vi "dfd_FXP Direct IIR II Transposed with IS.vi"(6 "state in":i64[](array[numeric]), 7 "quantizers":T5[](array[typedef]) {"source" items=["Coef a/k"=0, "Coef b/v"=7, "Input"=1, "Output"=2, "Multiplicand"=3, "Product"=4, "Sum"=5, "Delay"=6, "Gain"=8]}, 8 "filtering statistics in":T4(array[cluster]) {"statistics information"."min value" format="%.2f"; "statistics information"."max value" format="%.2f"; "Quantizer Source" items=["Coefficients a/k"=0, "Coefficients b/v"=7, "Input"=1, "Output"=2, "Multiplicand"=3, "Product"=4, "Sum"=5, "Delay"=6]}, 9 "coef a":T7, 10 "coef b":T7, 11 "X":T7) -> (0 "filtering statistics out":T4(array[cluster]) {"statistics information"."min value" format="%.2f"; "statistics information"."max value" format="%.2f"; "Quantizer Source" items=["Coefficients a/k"=0, "Coefficients b/v"=7, "Input"=1, "Output"=2, "Multiplicand"=3, "Product"=4, "Sum"=5, "Delay"=6]}, 3 "filtered X":T7, 4 "state out":i64[](array[numeric]))   [LabVIEW 2017, in "NI_DigFilter_FXP.lvlib"]
uses:
  <vilib>/addons/Digital Filter Design/NI_DigFilter_FXP.lvlib
  <vilib>/addons/Digital Filter Design/_Objects.llb/dfd_DFXP Data Type (vector).ctl
  <vilib>/addons/Digital Filter Design/_Objects.llb/dfd_DFXP Operation Parameter.ctl
  <vilib>/addons/Digital Filter Design/_Objects.llb/dfd_Internal Quantization Srcs.ctl
  <vilib>/addons/Digital Filter Design/_Objects.llb/DFD Quantization Sources.ctl
  <vilib>/addons/Digital Filter Design/_Objects.llb/DFD FXP Statistics Data.ctl
  <vilib>/addons/Digital Filter Design/_Objects.llb/dfd_DFXP Data Type (scaler).ctl
  <vilib>/addons/Digital Filter Design/NI_DigFilterLicensed.lvlib
panel:
  in  "DFXP Value":T1={"value"=0, "wl"=0, "iwl"=0, "Signed"=TRUE} {"value" format="%.0x"}
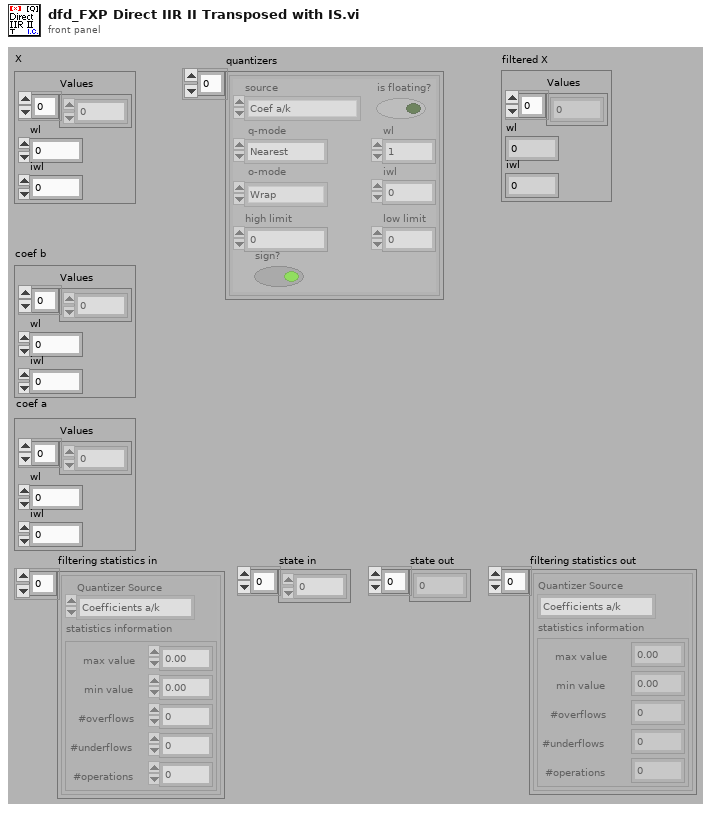
[diagram p1: front panel]
types:
  T1 = typedef "dfd_DFXP Data Type (scaler).ctl" = cluster{"value":i64, "wl":i16, "iwl":i16, "Signed":bool}
  T2 = typedef "NI_DigFilterLicensed.lvlib/DFD Quantization Sources.ctl" = u16
  T3 = typedef "NI_DigFilterLicensed.lvlib/DFD FXP Statistics Data.ctl" = cluster{"max value":ext, "min value":ext, "#overflows":i32, "#underflows":i32, "#operations":i32}
  T4 = cluster{"Quantizer Source":T2, "statistics information":T3}[]
  T5 = typedef "dfd_DFXP Operation Parameter.ctl" = cluster{"source":T6, "is floating?":bool, "o-mode":enum16{"Saturation", "Wrap"}, "q-mode":enum16{"Nearest", "Truncation"}, "wl":i16, "high limit":i64, "low limit":i64, "iwl":i16, "sign?":bool}
  T6 = typedef "NI_DigFilterLicensed.lvlib/dfd_Internal Quantization Srcs.ctl" = u16
  T7 = typedef "dfd_DFXP Data Type (vector).ctl" = cluster{"Values":i64[], "wl":i16, "iwl":i16}
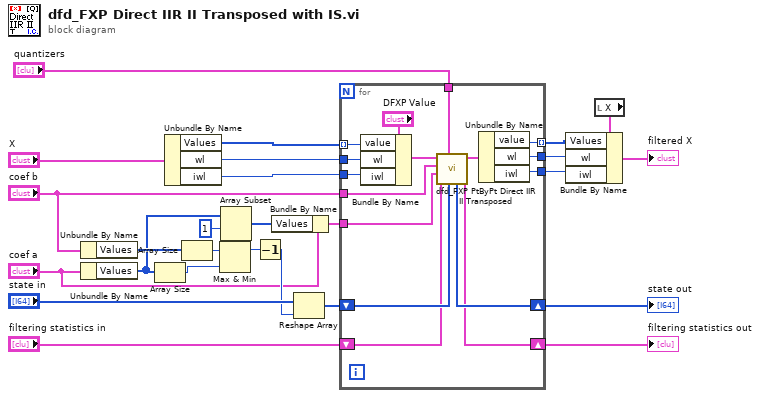
[diagram p0: block diagram]
diagram:
  n1 = Unbundle By Name("coef b") -> ("Values"=w11:i64[])
  n2 = Unbundle By Name("coef a") -> ("Values"=w10:i64[])
  n3 = Array Size(array=w10) -> (size(s)=w24:i32)
  n4 = Unbundle By Name("X") -> ("Values"=w7:i64[], "wl"=w6:i16, "iwl"=w5:i16)
  n5 = Array Size(array=w11) -> (size(s)=w23:i32)
  n6 = Max & Min(x=w23, y=w24) -> (max(x,y)=w21:i32)  [unwired: 1 out]
  n7 = Array Subset(array=w10, index=1) -> (w19:i64[])  [unwired: 1 in]
  n8 = Decrement(x=w21) -> (x-1=w14:i32)
  n9 = Bundle By Name(cluster="coef a", "Values"=w19) -> (w9:T7)
  n10 = Reshape Array("state in", w14) -> (w22:i64[])
  n11 = for {
    tunnel: w7 -> [w42] mode=indexing
    shift-right: [w36] -> w18
    shift-left: w22 -> [w37]
    tunnel: w9 -> [w39]
    tunnel: "coef b" -> [w40]
    tunnel: [w29] -> w16 mode=indexing
    tunnel: "quantizers" -> [w38]
    shift-right: [w34] -> w12
    shift-left: "filtering statistics in" -> [w35]
    tunnel: w6 -> [w31]
    tunnel: w5 -> [w30]
    tunnel: [w28] -> w2
    tunnel: [w27] -> w1
    n12 = Bundle By Name(cluster="DFXP Value", "value"=w42, "wl"=w31, "iwl"=w30) -> (w33:T1)
    n13 = call <vilib>:"dfd_FXP PtByPt Direct IIR II Transposed.vi"("state in"=w37, "quantizers"=w38, "filtering statistics in"=w35, "coef a[1..N]"=w39, "coef b[0..M]"=w40, "x"=w33) -> ("filtering statistics out"=w34:T4, "filtered x"=w41:T1, "state out"=w36:i64[])  [unwired: 3 out]
    n14 = Unbundle By Name(w41) -> ("value"=w29:i64, "wl"=w28:i16, "iwl"=w27:i16)
  }
  "state out" <- w18
  "filtering statistics out" <- w12
  n15 = local read "X"() -> (w3:T7)
  n16 = Bundle By Name(cluster=w3, "Values"=w16, "wl"=w2, "iwl"=w1) -> (→"filtered X":T7)
